vi "demo-edit-command.vi"() -> ()   [LabVIEW 2014]
uses:
  <vilib>/Plasmionique/MB Master/MB_Master_Serial/MB_Master_Serial.lvclass
panel:
  in  "stop":bool
  in  "execute command":bool
  in  "read command":bool
  in  "apply command":bool
  in  "command index":u16
  in  "command":T1={"type"=enum."abs_move", "position"=10.0, "velocity"=100.0, "acc"=3000.0, "dec"=3000.0, "band"=0.1, "push force"=30.0, "push distance"=30.0, "delay time"=500, "next command index"=-1}
  in  "save command":bool
  out "current position":dbl(slide) scale=0.0..95.0
  in  "baud rate (bps)":u32=9600
  in  "VISA Resource":refnum<visa-resource-name>
  in  "stop":bool
  in  "go home":bool
  out "errorCode":i32
  in  "servo":bool=TRUE
  in  "reset error":bool
  in  "axisNo":i32
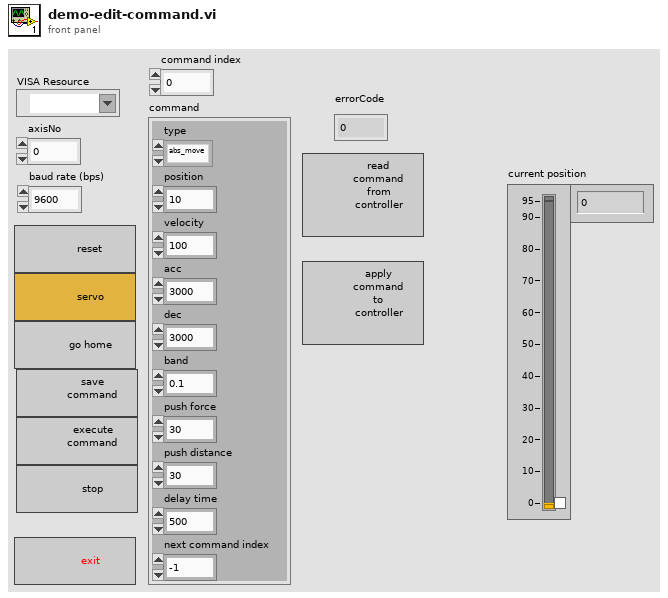
[diagram p1: front panel]
types:
  T1 = cluster{"type":enum16{"none", "go_home", "delay", "abs_move", "push", "inc_move"}, "position":dbl, "velocity":dbl, "acc":dbl, "dec":dbl, "band":dbl, "push force":dbl, "push distance":dbl, "delay time":i32, "next command index":i32}
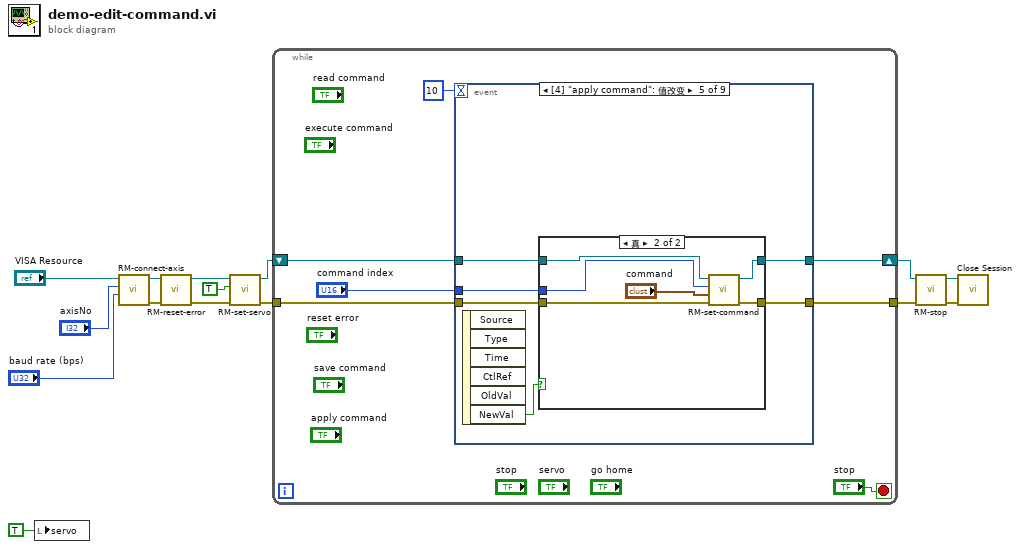
[diagram p0: block diagram]
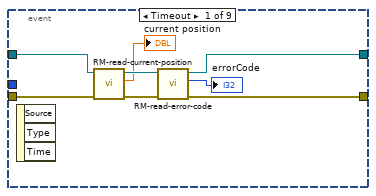
[diagram p2: hidden frame]
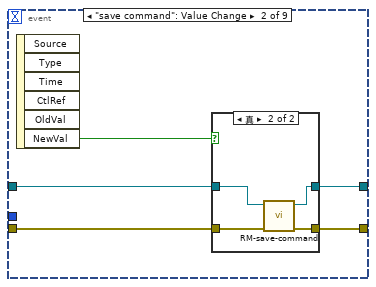
[diagram p3: hidden frame]
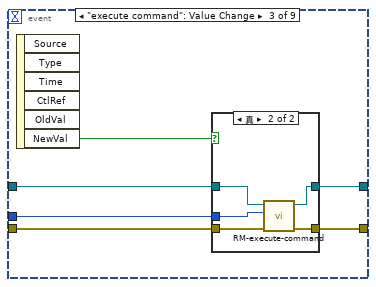
[diagram p5: hidden frame]
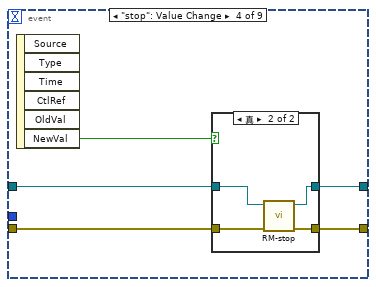
[diagram p7: hidden frame]
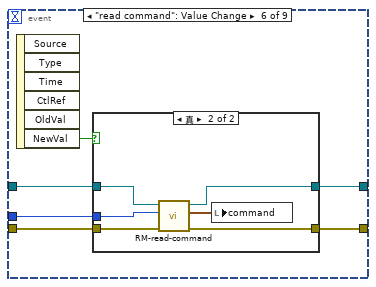
[diagram p10: hidden frame]
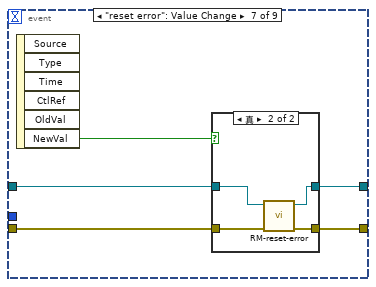
[diagram p12: hidden frame]
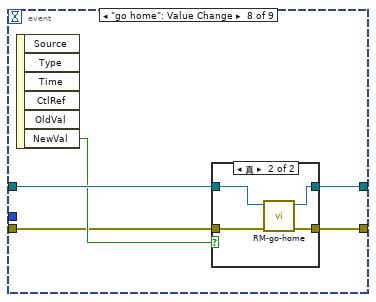
[diagram p14: hidden frame]
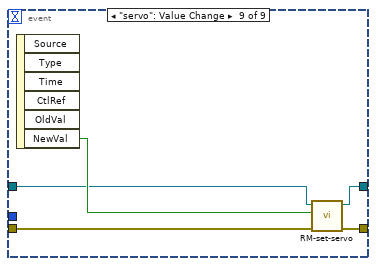
[diagram p16: hidden frame]
diagram:
  n1 = local write "servo"(TRUE ("servo")) -> ()
  n2 = call "RM-connect-axis.vi"("baud rate (bps)"="baud rate (bps)", "axisNo"="axisNo", "VISA引用句柄输入"="VISA Resource") -> ("Error out"=w8:errorcluster, "MB_Master_Serial输出"=w9:refnum<class "MB_Master_Serial.lvclass">)  [unwired: 7 in]
  n3 = call "RM-reset-error.vi"("错误输入（无错误）"=w8, "MB_Master_Serial输入"=w9) -> ("错误输出"=w10:errorcluster, "MB_Master_Serial输出"=w11:refnum<class "MB_Master_Serial.lvclass">)  [unwired: 8 in]
  n4 = call "RM-set-servo.vi"("error in (no error)"=w10, "servo-on?"=TRUE, "MB_Master_Serial输入"=w11) -> ("error out"=w2:errorcluster, "MB_Master_Serial输出"=w1:refnum<class "MB_Master_Serial.lvclass">)  [unwired: 7 in]
  n5 = while {
    shift-right: [w20] -> w7
    shift-left: w1 -> [w21]
    tunnel: [w18] -> w4
    tunnel: w2 -> [w17]
    stop <- "stop" stop-if-true
    n6 = event shown="[4] \"apply command\": 值改变" {
      selector: _ -> [_ _ _ _ _ _ _ _ _]
      dyn-events: _ -> [_ _ _ _ _ _ _ _ _]
      timeout: 10 -> [_ _ _ _ _ _ _ _ _]
      tunnel: w21 -> [w30 w35 w46 w58 w71 w84 w96 w109 w119]
      tunnel: [w25 w32 w43 w56 w69 w83 w97 w108 w118] -> w20
      tunnel: [w26 w33 w42 w55 w68 w82 w95 w106 w117] -> w18
      tunnel: w17 -> [w29 w34 w45 w57 w70 w85 w94 w105 w116]
      tunnel: "command index" -> [_ _ w44 _ w66 w81 _ _ _]
      event Timeout {
        n7 = event-data() -> ()  [unwired: 1 in, 3 out]
        n8 = call "RM-read-current-position.vi"("错误输入（无错误）"=w29, "MB_Master_Serial输入"=w30) -> ("错误输出"=w27:errorcluster, "数值"=→"current position":dbl, "MB_Master_Serial输出"=w28:refnum<class "MB_Master_Serial.lvclass">)  [unwired: 7 in]
        n9 = call "RM-read-error-code.vi"("错误输入（无错误）"=w27, "MB_Master_Serial输入"=w28) -> ("错误输出"=w26:errorcluster, "error_code"=→"errorCode":i32, "MB_Master_Serial输出"=w25:refnum<class "MB_Master_Serial.lvclass">)  [unwired: 7 in]
      }
      event "save command": Value Change {
        n10 = event-data() -> ("NewVal"=w31:bool)  [unwired: 1 in, 5 out]
        n11 = case shown="真" w31 {
          tunnel: w35 -> [w37 w41]
          tunnel: w34 -> [w36 w40]
          tunnel: [w36 w39] -> w33
          tunnel: [w37 w38] -> w32
          frame False {
          }
          frame True {
            n12 = call "RM-save-command.vi"("错误输入（无错误）"=w40, "MB_Master_Serial输入"=w41) -> ("错误输出"=w39:errorcluster, "MB_Master_Serial输出"=w38:refnum<class "MB_Master_Serial.lvclass">)  [unwired: 8 in]
          }
        }
      }
      event "execute command": Value Change {
        n13 = event-data() -> ("NewVal"=w47:bool)  [unwired: 1 in, 5 out]
        n14 = case shown="真" w47 {
          tunnel: w46 -> [w49 w54]
          tunnel: w45 -> [w48 w53]
          tunnel: w44 -> [_ w52]
          tunnel: [w49 w51] -> w43
          tunnel: [w48 w50] -> w42
          frame False {
          }
          frame True {
            n15 = call "RM-execute-command.vi"("error in (no error)"=w53, "command index"=w52, "MB_Master_Serial输入"=w54) -> ("error out"=w50:errorcluster, "MB_Master_Serial输出"=w51:refnum<class "MB_Master_Serial.lvclass">)  [unwired: 7 in]
          }
        }
      }
      event "stop": Value Change {
        n16 = event-data() -> ("NewVal"=w59:bool)  [unwired: 1 in, 5 out]
        n17 = case shown="真" w59 {
          tunnel: w58 -> [w61 w65]
          tunnel: w57 -> [w60 w64]
          tunnel: [w61 w63] -> w56
          tunnel: [w60 w62] -> w55
          frame False {
          }
          frame True {
            n18 = call "RM-stop.vi"("error in (no error)"=w64, "MB_Master_Serial输入"=w65) -> ("error out"=w62:errorcluster, "MB_Master_Serial输出"=w63:refnum<class "MB_Master_Serial.lvclass">)  [unwired: 8 in]
          }
        }
      }
      event "apply command": Value Change {
        n19 = event-data() -> ("NewVal"=w67:bool)  [unwired: 1 in, 5 out]
        n20 = case shown="真" w67 {
          tunnel: w71 -> [w73 w78]
          tunnel: w70 -> [w72 w77]
          tunnel: [w73 w76] -> w69
          tunnel: [w72 w75] -> w68
          tunnel: w66 -> [_ w74]
          frame False {
          }
          frame True {
            n21 = call "RM-set-command.vi"("error in (no error)"=w77, "command"="command", "command index"=w74, "MB_Master_Serial输入"=w78) -> ("error out"=w75:errorcluster, "MB_Master_Serial输出"=w76:refnum<class "MB_Master_Serial.lvclass">)  [unwired: 6 in]
          }
        }
      }
      event "read command": Value Change {
        n22 = event-data() -> ("NewVal"=w80:bool)  [unwired: 1 in, 5 out]
        n23 = case shown="真" w80 {
          tunnel: w85 -> [w86 w90]
          tunnel: w84 -> [w87 w93]
          tunnel: [w87 w92] -> w83
          tunnel: [w86 w91] -> w82
          tunnel: w81 -> [_ w89]
          frame False {
          }
          frame True {
            n24 = call "RM-read-command.vi"("error in (no error)"=w90, "command index"=w89, "MB_Master_Serial输入"=w93) -> ("error out"=w91:errorcluster, "command"=w88:T1, "MB_Master_Serial输出"=w92:refnum<class "MB_Master_Serial.lvclass">)  [unwired: 6 in]
            n25 = local write "command"(w88) -> ()
          }
        }
      }
      event "reset error": Value Change {
        n26 = event-data() -> ("NewVal"=w98:bool)  [unwired: 1 in, 5 out]
        n27 = case shown="真" w98 {
          tunnel: [w100 w103] -> w97
          tunnel: w96 -> [w100 w104]
          tunnel: [w99 w102] -> w95
          tunnel: w94 -> [w99 w101]
          frame False {
          }
          frame True {
            n28 = call "RM-reset-error.vi"("错误输入（无错误）"=w101, "MB_Master_Serial输入"=w104) -> ("错误输出"=w102:errorcluster, "MB_Master_Serial输出"=w103:refnum<class "MB_Master_Serial.lvclass">)  [unwired: 8 in]
          }
        }
      }
      event "go home": Value Change {
        n29 = event-data() -> ("NewVal"=w107:bool)  [unwired: 1 in, 5 out]
        n30 = case shown="真" w107 {
          tunnel: w109 -> [w111 w115]
          tunnel: [w111 w114] -> w108
          tunnel: [w110 w113] -> w106
          tunnel: w105 -> [w110 w112]
          frame False {
          }
          frame True {
            n31 = call "RM-go-home.vi"("error in (no error)"=w112, "MB_Master_Serial输入"=w115) -> ("error out"=w113:errorcluster, "MB_Master_Serial输出"=w114:refnum<class "MB_Master_Serial.lvclass">)  [unwired: 8 in]
          }
        }
      }
      event "servo": Value Change {
        n32 = event-data() -> ("NewVal"=w120:bool)  [unwired: 1 in, 5 out]
        n33 = call "RM-set-servo.vi"("error in (no error)"=w116, "servo-on?"=w120, "MB_Master_Serial输入"=w119) -> ("error out"=w117:errorcluster, "MB_Master_Serial输出"=w118:refnum<class "MB_Master_Serial.lvclass">)  [unwired: 7 in]
      }
    }
  }
  n34 = call "RM-stop.vi"("error in (no error)"=w4, "MB_Master_Serial输入"=w7) -> ("error out"=w5:errorcluster, "MB_Master_Serial输出"=w6:refnum<class "MB_Master_Serial.lvclass">)  [unwired: 8 in]
  n35 = call-dynamic "Close Session.vi"("error in (no error)"=w5, "MB_Serial session"=w6) -> ()  [unwired: 9 in, 1 out]
